vi "Initialize Reference Lasers.vi"(8 "error in (no error)":errorcluster, 11 "Range Controller Actor in":refnum<class "Range Controller Actor.lvclass">) -> (0 "error out":errorcluster, 3 "Range Controller Actor out":refnum<class "Range Controller Actor.lvclass">)   [LabVIEW 2018, in "Range Controller.lvlib" / "Range Controller Actor.lvclass"]
uses:
  Range Controller Actor.lvclass
  C:/Program Files (x86)/National Instruments/LabVIEW 2018/vi.lib/ActorFramework/Actor/Actor.lvclass
  Range Controller Actor.lvclass/Range Controller Actor.ctl
  DLS Laser Actor/FLS Laser Actor.lvclass
  <vilib>/ActorFramework/Actor/Actor.lvclass
  DLS Laser Actor/DLS Laser Actor Messages/Initialize DLS Laser Msg/Initialize FLS Laser Msg.lvclass
types:
  T1 = typedef "MWWL Verification.lvlib/Ranges Refnum.ctl" = refnum<vi>
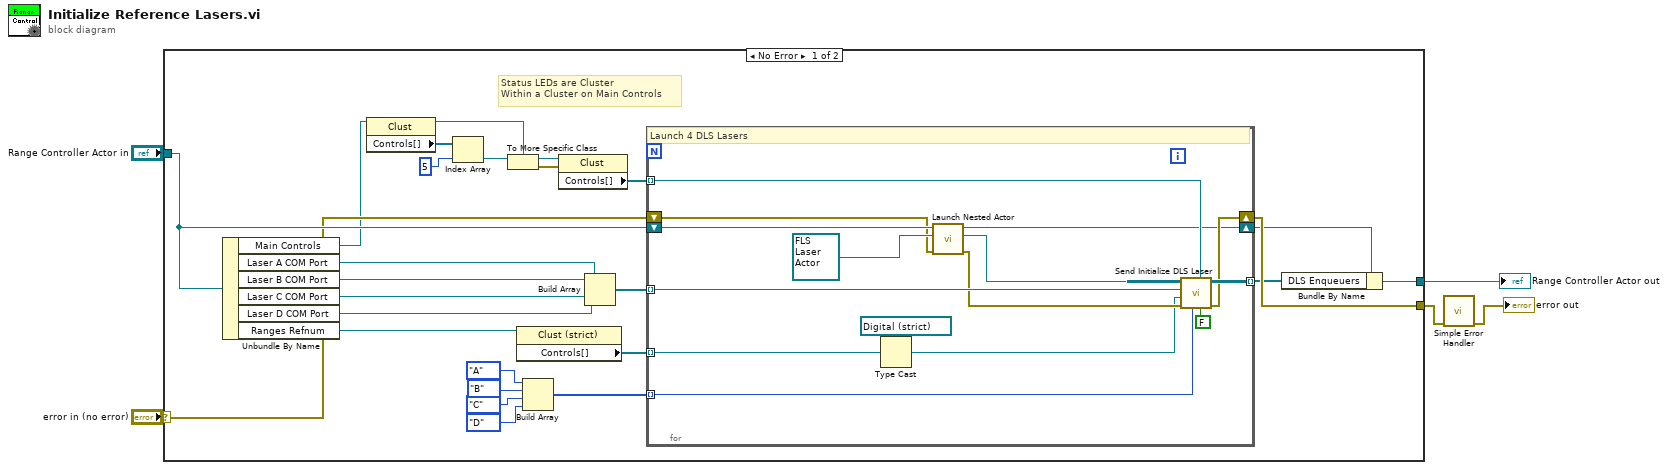
[diagram p0: block diagram]
diagram:
  n1 = case shown="No Error" "error in (no error)" {
    selector: "error in (no error)" -> [w17 w48]
    tunnel: [w26 w48] -> w2
    tunnel: [w18 w47] -> w4
    tunnel: "Range Controller Actor in" -> [w20 w47]
    frame No Error {
      # "Status LEDs are Cluster \nWithin a Cluster on Main Controls"
      n2 = Unbundle By Name(w20) -> ("Main Controls"=w10:refnum<vi>, "Laser A COM Port"=w28:refnum<visa-resource-name>, "Laser B COM Port"=w29:refnum<visa-resource-name>, "Laser C COM Port"=w30:refnum<visa-resource-name>, "Laser D COM Port"=w31:refnum<visa-resource-name>, "Ranges Refnum"=w7:T1)
      n3 = property class="Clust"(reference=w10) -> (reference out=w11:refnum<vi>, "Controls[]"=w14:refnum<vi>[])  [unwired: 1 in, 1 out]
      n4 = Index Array(array=w14, index=5) -> (element=w13:refnum<vi>)
      n5 = To More Specific Class(target class=w11, reference=w13) -> (specific class reference=w15:refnum<vi>, error out=w16:errorcluster)  [unwired: 1 in]
      n6 = property class="Clust (strict)"(reference=w7) -> ("Controls[]"=w8:refnum<vi>[])  [unwired: 1 in, 2 out]
      n7 = Build Array(enum16{"A", "B", "C", "D"}."A" ("DLS Laser ID (A,B,C or D)"), enum16{"A", "B", "C", "D"}."B" ("DLS Laser ID (A,B,C or D)"), enum16{"A", "B", "C", "D"}."C" ("DLS Laser ID (A,B,C or D)"), enum16{"A", "B", "C", "D"}."D" ("DLS Laser ID (A,B,C or D)")) -> (w21:enum16{"A", "B", "C", "D"}[])
      n8 = property class="Clust"(reference=w15, error in=w16) -> ("Controls[]"=w9:refnum<vi>[])  [unwired: 2 out]
      n9 = Build Array(w28, w29, w30, w31) -> (w27:refnum<visa-resource-name>[])
      n10 = for {
        tunnel: w27 -> [w44] mode=indexing
        tunnel: w21 -> [w36] mode=indexing
        tunnel: [w40] -> w19 mode=indexing
        tunnel: w9 -> [w34] mode=indexing
        tunnel: w8 -> [w33] mode=indexing
        shift-right: [w32] -> w6
        shift-left: w20 -> [w43]
        shift-right: [w42] -> w26
        shift-left: w17 -> [w39]
        # "Launch 4 DLS Lasers"
        n11 = Type Cast(type=refnum<vi> refnum ("DLS Range Refnum"), x=w33) -> (*(type *) &x=w37:refnum<vi>)
        n12 = call <vilib>:"Launch Nested Actor.vi"("error in (no error)"=w39, "Nested Actor"=refnum<class "FLS Laser Actor.lvclass"> refnum ("DLS Laser Actor.lvlib:DLS Laser Actor"), "Caller Actor in"=w43) -> ("error out"=w41:errorcluster, "Nested Actor's Enqueuer"=w45:refnum<class "Message Enqueuer.lvclass">, "Caller Actor out"=w32:refnum<class "Range Controller Actor.lvclass">)  [unwired: 6 in]
        n13 = call "Send Initialize DLS Laser.vi"("Fault?"=FALSE, "DLS Status LEDs Refnum"=w34, "DLS Laser ID (A,B,C or D)"=w36, "error in (no error)"=w41, "DLS Range Refnum"=w37, "DLS COM Port"=w44, "Message Enqueuer in"=w45) -> ("error out"=w42:errorcluster, "Message Enqueuer out"=w40:refnum<class "Message Enqueuer.lvclass">)  [unwired: 3 in]
      }
      n14 = Bundle By Name(cluster=w6, "DLS Enqueuers"=w19) -> (w18:refnum<class "Range Controller Actor.lvclass">)
    }
    frame Error {
    }
  }
  "Range Controller Actor out" <- w4
  n15 = call <vilib>:"Simple Error Handler.vi"("error in (no error)"=w2) -> ("error out"=→"error out":errorcluster)  [unwired: 4 in, 4 out]
